vi "Index Arrays for specific Loop.vi"(6 "Array of Indeces":u32[](array[numeric]), 8 "error in (no error)":errorcluster, 9 "Type code Array":i32[](array[numeric]), 10 "Array of SV Refnums":refnum<k21>[](array[refnum]), 11 "Names":string[](array[string])) -> (0 "error out":errorcluster, 1 "Indexed Type Code":i32[](array[numeric]), 2 "Indexed SV Refnums":refnum<k21>[](array[refnum]), 3 "Indexed Names":string[](array[string]))   [LabVIEW 2014]
doc: "<B>Copyright</B>: (c) MHWirth 2015.\n\nThis VI indexes 3 input arrays based on the Array of Indeces."
uses:
  Index Arrays - sv refnum.vi
  Index Arrays - string.vi
  Index Arrays - I32.vi
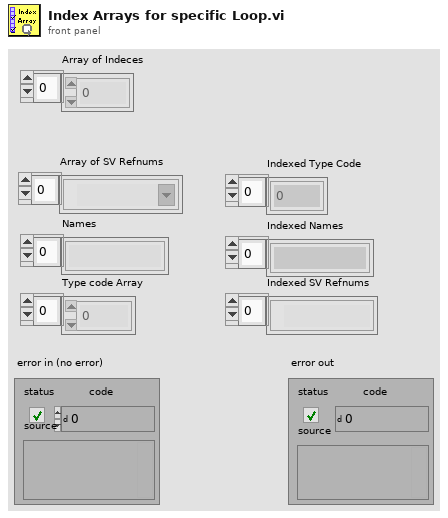
[diagram p1: front panel]
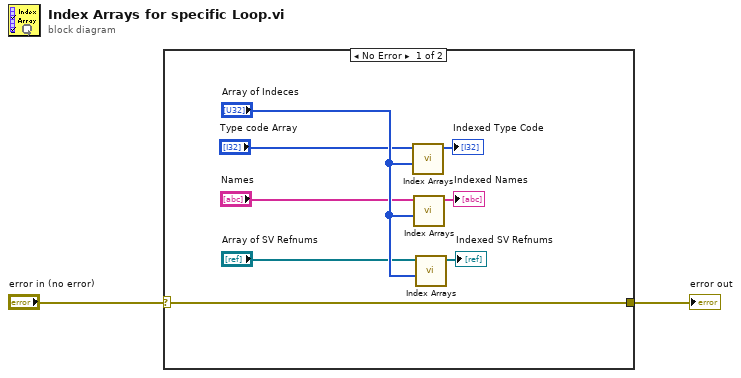
[diagram p0: block diagram]
diagram:
  n1 = case shown="No Error" "error in (no error)" {
    selector: "error in (no error)" -> [w10 w11]
    tunnel: [w10 w11] -> w1
    frame No Error {
      n2 = call-poly "Index Arrays.vi"("Index array"="Array of Indeces", "Array in"="Type code Array") -> ("Array out"=→"Indexed Type Code":i32[])  [unwired: 9 in]
      n3 = call-poly "Index Arrays.vi"("Index array"="Array of Indeces", "Array in"="Names") -> ("Array out"=→"Indexed Names":string[])  [unwired: 9 in]
      n4 = call-poly "Index Arrays.vi"("Index array"="Array of Indeces", "Array in"="Array of SV Refnums") -> ("Array out"=→"Indexed SV Refnums":refnum<k21>[])  [unwired: 9 in]
    }
    frame Error {
    }
  }
  "error out" <- w1
